vi "OpenCasperDrve.vi"(5 "ClimbRev":dbl, 7 "Encoder Ticks Per Rev":dbl, 8 "error in (no error)":errorcluster, 9 "PID (Distance)":T1, 10 "PID (Speed)":T1, 11 "Drive Subsystem Global in":T2) -> (0 "error out":errorcluster, 1 "RobotDriveRef":T6={"RobotDriveDevRef"={"DevStatus"={"status"=FALSE, "code"=0, "source"=""}, "Motors[]"=[], "Square Inputs"=FALSE, "Max Output"=0.0}, "Control Mode"=enum."Percent VBus", "Motor Settings"={"Wheel Radius"=0.0, "Encoder Ticks Per Rev"=0.0, "Gear Ratio"=0.0, "ClimbRev"=0.0}, "Default Control Mode"=enum."Unchanged / Invalid"}, 2 "Control Mode":T5, 3 "Drive Subsystem Global out":T2)   [LabVIEW 2015]
uses:
  Advanced Drive VIs/RobotDrive Type Def.ctl
  <vilib>/Rock Robotics/WPI/MotorControl/WPI_MotorControlDeviceRef.ctl
  <vilib>/Rock Robotics/WPI/MotorControl/WPI_MotorControlType.ctl
  <vilib>/Rock Robotics/SystemInterfaces/DIO/FPGA_DIOPWMChannel.ctl
  <vilib>/Rock Robotics/WPI/PWM/WPI_PWMDeadband.ctl
  <vilib>/Rock Robotics/WPI/CAN/Jaguar/SubVIs/WPI_CANJaguar_ControlMode.ctl
  <vilib>/Rock Robotics/WPI/CAN/TalonSRX/WPI_CANTalonSRX_APIControlMode.ctl
  Advanced Drive VIs/Drive Motor Settings.ctl
  LED Lights/Drive Global Type Def.ctl
  LED Lights/Master Slave Drive Motors Type Def.ctl
  LED Lights/Motor Global Type Def.ctl
  Advanced Drive VIs/PID Type Def.ctl
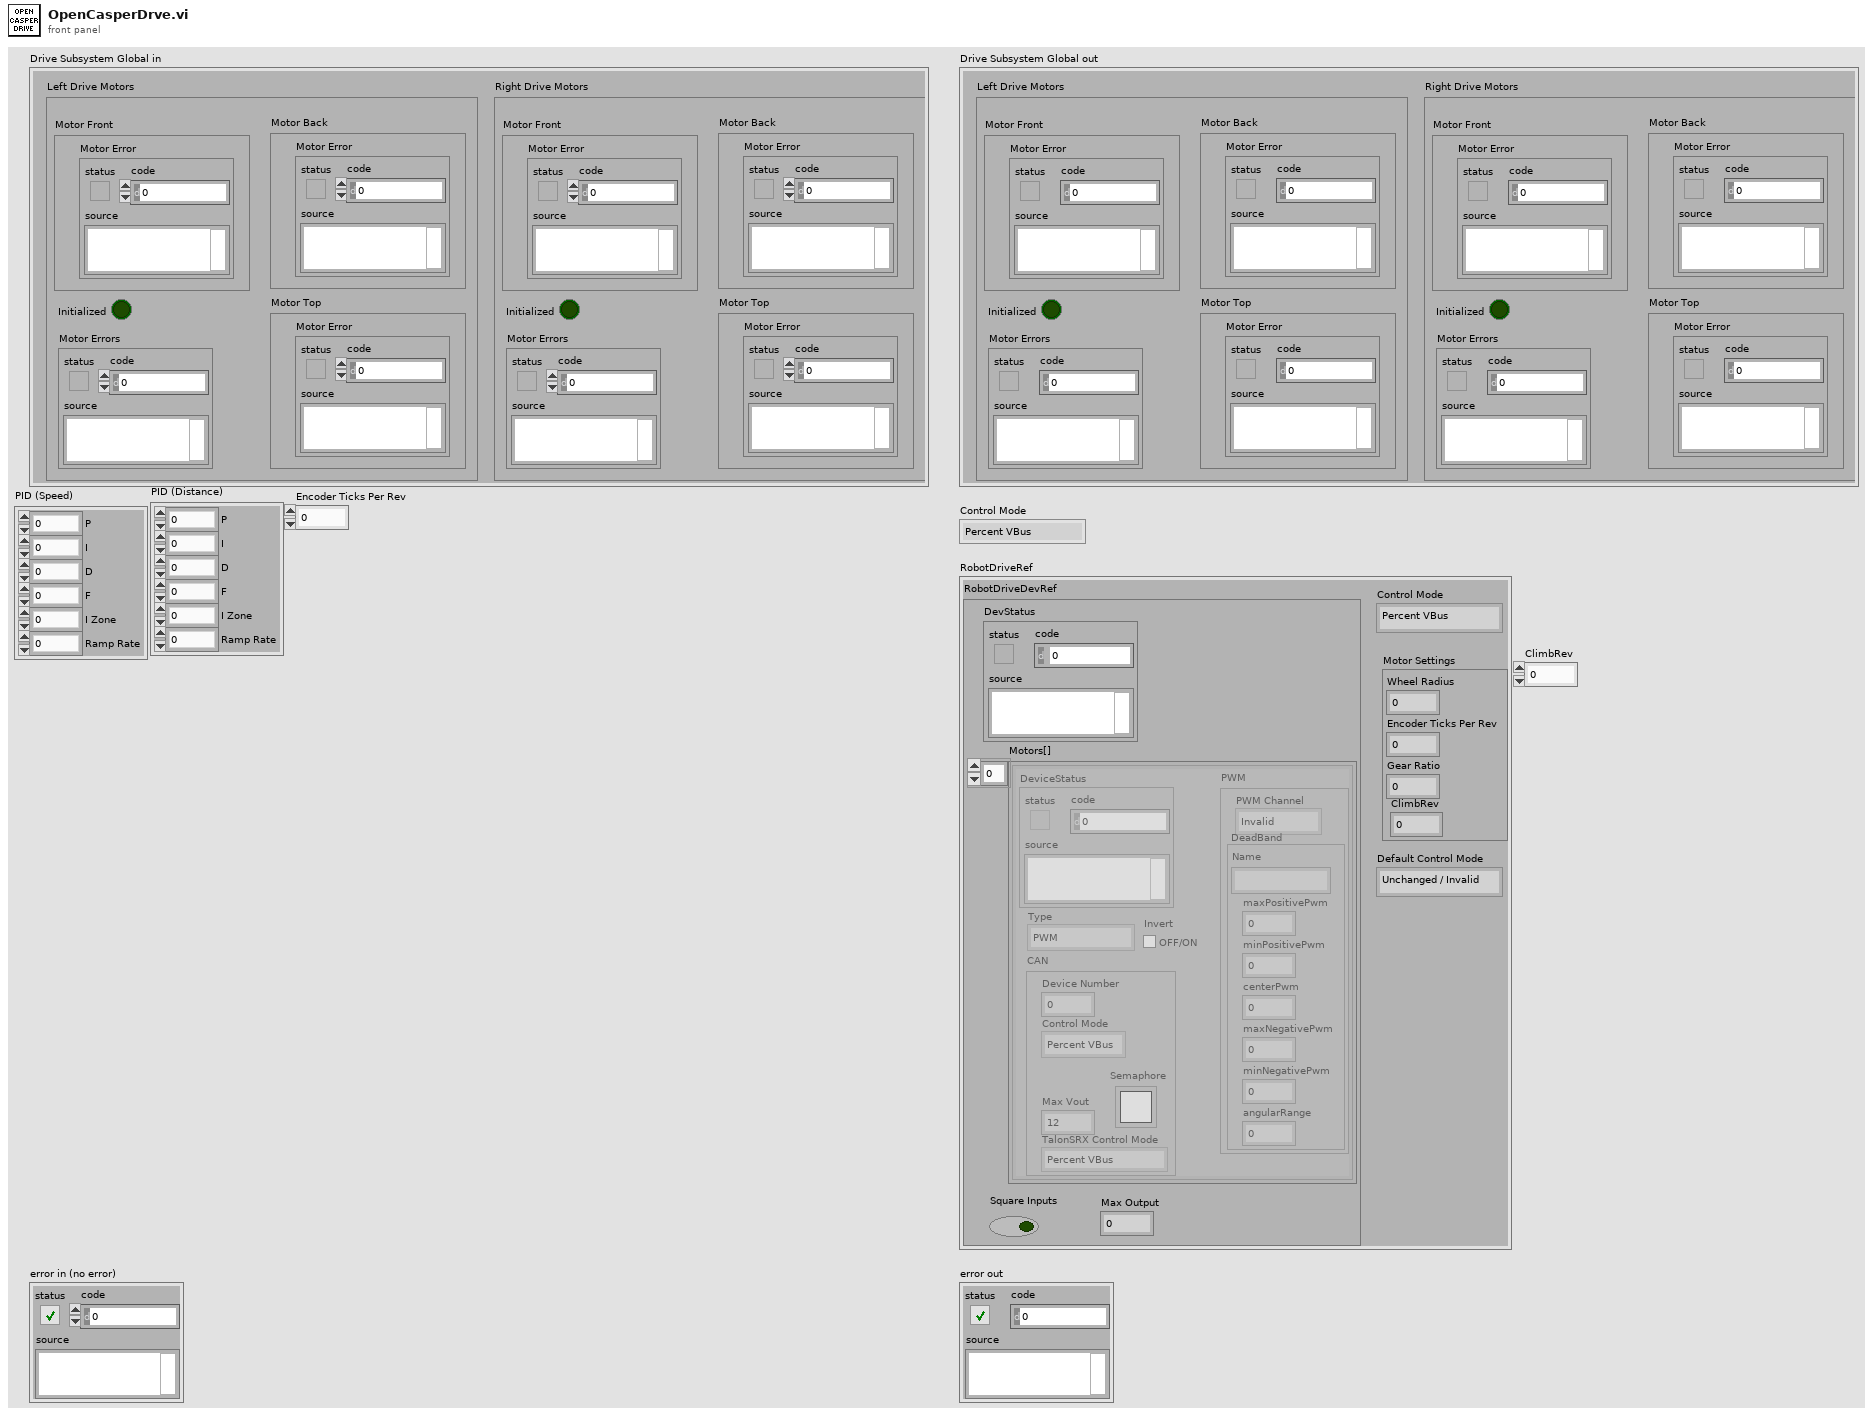
[diagram p1: front panel]
types:
  T1 = typedef "PID Type Def.ctl" = cluster{"P":dbl, "I":dbl, "D":dbl, "F":dbl, "I Zone":dbl, "Ramp Rate":dbl}
  T2 = typedef "Drive Global Type Def.ctl" = cluster{"Left Drive Motors":T3, "Right Drive Motors":T3}
  T3 = typedef "Master Slave Drive Motors Type Def.ctl" = cluster{"Motor Front":T4, "Motor Back":T4, "Motor Errors":errorcluster, "Motor Top":T4, "Initialized":bool}
  T4 = typedef "Motor Global Type Def.ctl" = cluster{"Motor Error":errorcluster}
  T5 = typedef "WPI_CANTalonSRX_APIControlMode.ctl" = enum8{"Percent VBus", "Speed", "Position", "Slave", "Unchanged / Invalid", "Voltage Compensation", "Current", "Motion Profile"}
  T6 = typedef "RobotDrive Type Def.ctl" = cluster{"RobotDriveDevRef":cluster{"DevStatus":errorcluster, "Motors[]":T7[], "Square Inputs":bool, "Max Output":dbl}, "Control Mode":T5, "Motor Settings":T13, "Default Control Mode":T5}
  T7 = typedef "WPI_MotorControlDeviceRef.ctl" = cluster{"DeviceStatus":errorcluster, "Type":T8, "PWM":cluster{"PWM Channel":T9, "DeadBand":T10}, "CAN":cluster{"Device Number":u8, "Control Mode":T11, "Semaphore":T12, "Max Vout":dbl, "TalonSRX Control Mode":T5}, "Invert":bool}
  T8 = typedef "WPI_MotorControlType.ctl" = enum16{"PWM", "CAN", "CANTalonSRX"}
  T9 = typedef "FPGA_DIOPWMChannel.ctl" = enum8{"PWM 0", "PWM 1", "PWM 2", "PWM 3", "PWM 4", "PWM 5", "PWM 6", "PWM 7", "PWM 8", "PWM 9", "PWM MXP 0", "PWM MXP 1", "PWM MXP 2", "PWM MXP 3", "PWM MXP 4", "PWM MXP 5", "PWM MXP 6", "PWM MXP 7", "PWM MXP 8", "PWM MXP 9", "Invalid"}
  T10 = typedef "WPI_PWMDeadband.ctl" = cluster{"Name":string, "maxPositivePwm":i32, "minPositivePwm":i32, "centerPwm":i32, "maxNegativePwm":i32, "minNegativePwm":i32, "angularRange":u16}
  T11 = typedef "WPI_CANJaguar_ControlMode.ctl" = enum8{"Percent VBus", "Current", "Speed", "Position", "Voltage"}
  T12 = typedef "Semaphore RefNum" = refnum<k1>
  T13 = typedef "Drive Motor Settings.ctl" = cluster{"Wheel Radius":dbl, "Encoder Ticks Per Rev":dbl, "Gear Ratio":dbl, "ClimbRev":dbl}
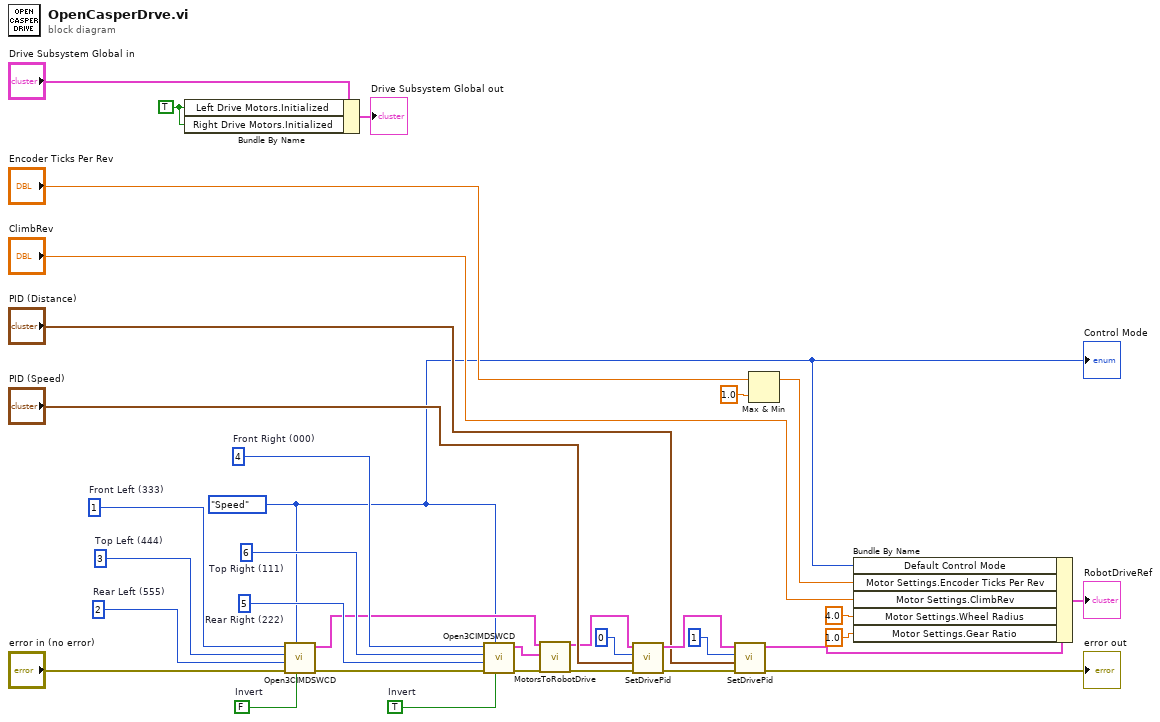
[diagram p0: block diagram]
diagram:
  w32 = TRUE
  w29 = TRUE  # Invert
  w25 = FALSE  # Invert
  w27 = u8 6  # Top Right (111)
  w28 = u8 5  # Rear Right (222)
  w26 = u8 4  # Front Right (000)
  w23 = u8 3  # Top Left (444)
  w24 = u8 2  # Rear Left (555)
  w22 = u8 1  # Front Left (333)
  w1 = WPI_CANTalonSRX_APIControlMode."Speed" ("Control Mode")
  n1 = Bundle By Name(cluster="Drive Subsystem Global in", "Left Drive Motors.Initialized"=w32, "Right Drive Motors.Initialized"=w32) -> (→"Drive Subsystem Global out":T2)
  n2 = call "Open3CIMDSWCD.vi"("Invert"=w25, "Control Mode"=w1, "error in (no error)"="error in (no error)", "Bottom Back"=w24, "Top Middle"=w23, "Bottom Front"=w22) -> ("error out"=w34:errorcluster, "CAN Talon SRX Ref"=w7:T7)  [unwired: 4 in]
  n3 = call "Open3CIMDSWCD.vi"("Invert"=w29, "Control Mode"=w1, "error in (no error)"=w34, "Bottom Back"=w28, "Top Middle"=w27, "Bottom Front"=w26) -> ("error out"=w5:errorcluster, "CAN Talon SRX Ref"=w6:T7)  [unwired: 4 in]
  n4 = call "MotorsToRobotDrive.vi"("Left"=w7, "Right"=w6, "error in"=w5) -> ("RobotDriveRef"=w8:T6, "error out"=w4:errorcluster)  [unwired: 15 in]
  n5 = call "SetDrivePid.vi"("error in (no error)"=w4, "PID"="PID (Speed)", "Profile Slot"=u8 0, "RobotDriveRef In"=w8) -> ("error out"=w18:errorcluster, "RobotDriveRef Out"=w19:T6)  [unwired: 6 in]
  n6 = call "SetDrivePid.vi"("error in (no error)"=w18, "PID"="PID (Distance)", "Profile Slot"=u8 1, "RobotDriveRef In"=w19) -> ("error out"=→"error out":errorcluster, "RobotDriveRef Out"=w13:T6)  [unwired: 6 in]
  n7 = Max & Min(x="Encoder Ticks Per Rev", y=1.0) -> (max(x,y)=w11:dbl)  [unwired: 1 out]
  n8 = Bundle By Name(cluster=w13, "Default Control Mode"=w1, "Motor Settings.Encoder Ticks Per Rev"=w11, "Motor Settings.ClimbRev"="ClimbRev", "Motor Settings.Wheel Radius"=4.0, "Motor Settings.Gear Ratio"=1.0) -> (→"RobotDriveRef":T6)
  "Control Mode" <- w1
